vi "Process.vi"(11 "Actor":refnum<class "Status Window.lvclass">) -> ()   [LabVIEW 2015, in "Status Window.lvclass"]
uses:
  Status Window.lvclass
  Re-use Libraries/Minimal Actor Framework/Actors/Base Actor/Actor/Front Panel State.ctl
  Re-use Libraries/Minimal Actor Framework/Actors/Base Actor/Actor/Actor.lvclass
  Re-use Libraries/Minimal Actor Framework/Messaging/Message/Message.lvclass
  Actors/Alarm Handler/API/Alarm Handler Actor API.lvclass
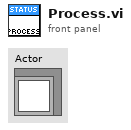
[diagram p1: front panel]
types:
  T1 = typedef "Actor.lvclass/Front Panel State.ctl" = enum32{"Invalid", "Standard", "Closed", "Hidden", "Minimized", "Maximized"}
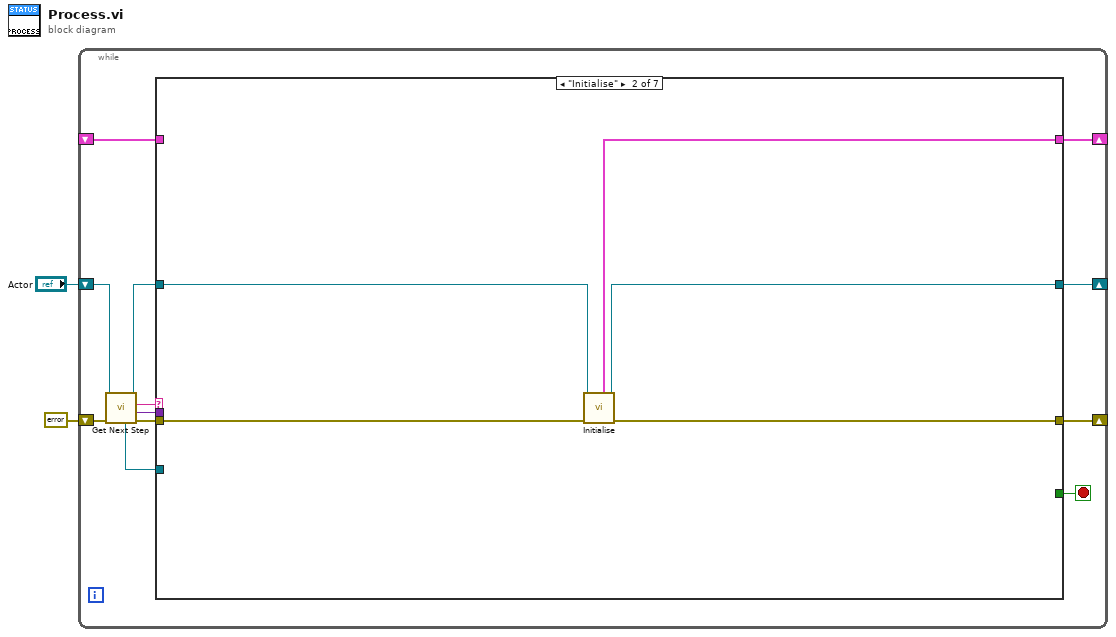
[diagram p0: block diagram]
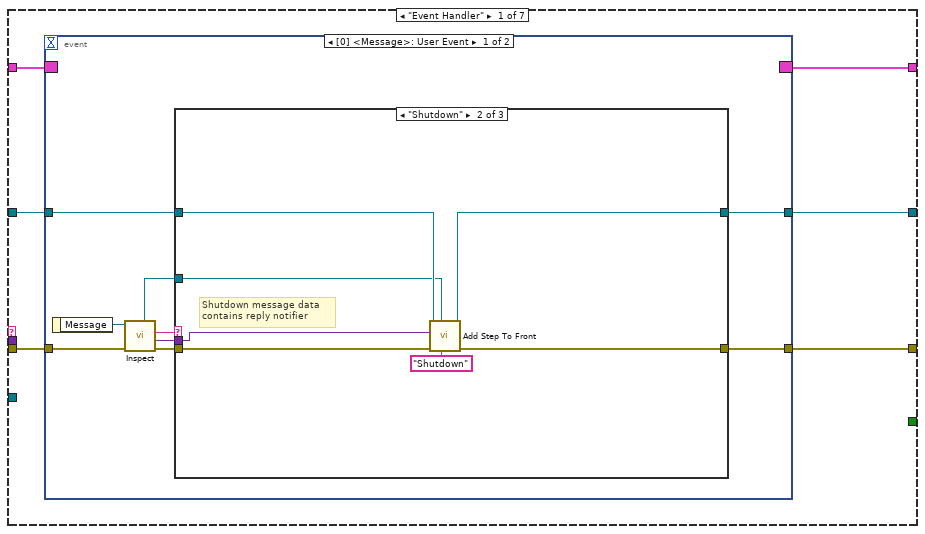
[diagram p2: hidden frame]
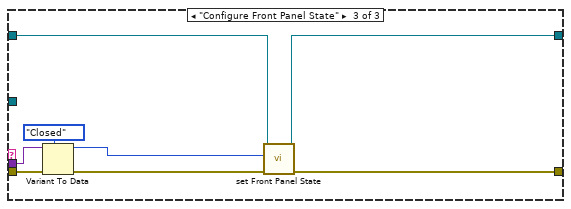
[diagram p4: hidden frame]
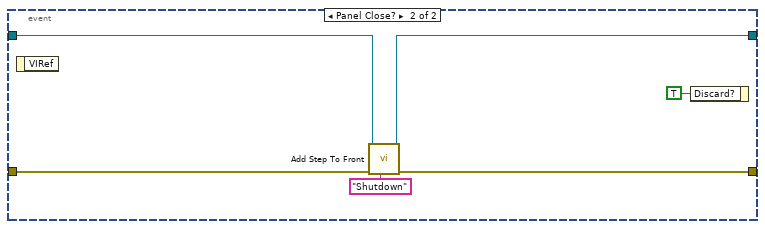
[diagram p5: hidden frame]
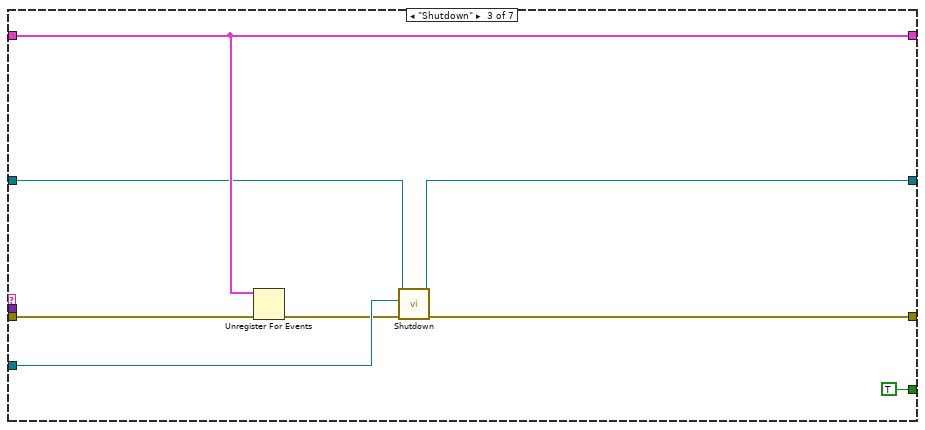
[diagram p6: hidden frame]
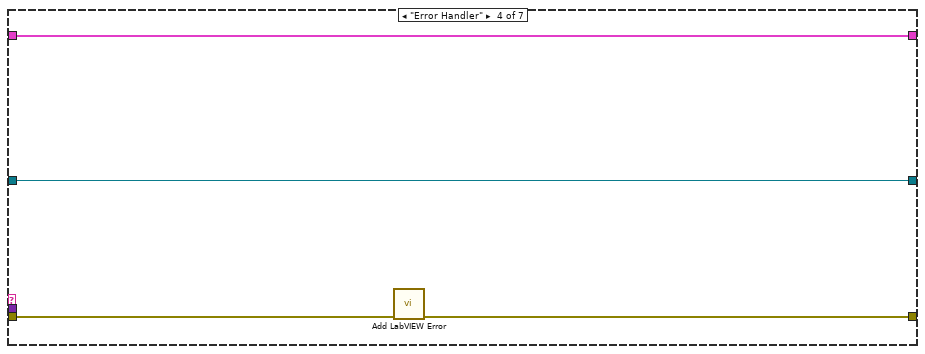
[diagram p7: hidden frame]
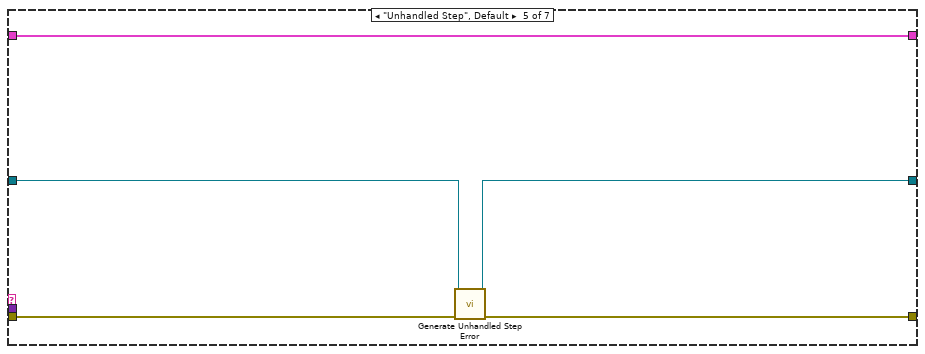
[diagram p8: hidden frame]
diagram:
  n1 = while {
    shift-right: [w5] -> _
    shift-left: "Actor" -> [w13]
    shift-right: [w10] -> _
    shift-left: _ -> [w9]
    shift-right: [w4] -> _
    shift-left: errorcluster {"status"=FALSE, "code"=0, "source"=""} ("error constant") -> [w7]
    stop <- w14 stop-if-true
    n2 = call-dynamic "Get Next Step.vi"("error in (no error)"=w7, "Actor in"=w13) -> ("error out"=w8:errorcluster, "Parameter"=w11:variant, "Step"=w6:string, "Actor out"=w12:refnum<class "Status Window.lvclass">, "Reply Channel"=w3:refnum<notifier>)  [unwired: 5 in]
    n3 = case shown="\"Initialise\"" w6 {
      tunnel: [_ _ TRUE _ _ _ _] -> w14
      tunnel: w12 -> [w20 w55 w63 w66 w73 w76 w78]
      tunnel: [w15 w53 w62 w66 w72 w76 w78] -> w5
      tunnel: w11 -> [_ _ _ _ _ _ _]
      tunnel: [w18 w57 w64 w69 w74 w77 w80] -> w10
      tunnel: w9 -> [w19 _ w64 w69 w74 w77 w80]
      tunnel: w8 -> [w17 w54 w60 w68 w71 w75 w79]
      tunnel: [w16 w56 w58 w67 w70 w75 w79] -> w4
      tunnel: w3 -> [_ _ w61 _ _ _ _]
      frame "Event Handler" {
        n4 = event shown="[0] <Message>: User Event" {
          selector: w19 -> [_ _]
          dyn-events: [_ _] -> w18
          timeout: _ -> [_ _]
          tunnel: w20 -> [w29 w48]
          tunnel: [w28 w47] -> w15
          tunnel: w17 -> [w26 w50]
          tunnel: [w27 w49] -> w16
          event User Event {
            n5 = event-data() -> ("Message"=w25:refnum<class "Message.lvclass">)  [unwired: 1 in]
            n6 = call "Inspect.vi"("error in (no error)"=w26, "Message in"=w25) -> ("error out"=w22:errorcluster, "Data"=w23:variant, "Name"=w24:string, "Reply Channel"=w21:refnum<notifier>)  [unwired: 5 in, 1 out]
            n7 = case shown="\"Shutdown\"" w24 {
              tunnel: w29 -> [w31 w38 w46]
              tunnel: [w31 w37 w45] -> w28
              tunnel: w22 -> [w30 w35 w42]
              tunnel: [w30 w34 w44] -> w27
              tunnel: w23 -> [_ w33 w43]
              tunnel: w21 -> [_ w32 _]
              frame Default {
              }
              frame "Shutdown" {
                # "Shutdown message data contains reply notifier"
                n8 = call-dynamic "Add Step To Front.vi"("Step Name"="Shutdown", "Reply Channel"=w32, "error in (no error)"=w35, "Parameter"=w33, "Actor in"=w38) -> ("error out"=w34:errorcluster, "Actor out"=w37:refnum<class "Status Window.lvclass">)  [unwired: 5 in]
              }
              frame "Configure Front Panel State" {
                n9 = Variant To Data(error in=w42, type=Front_Panel_State."Closed" ("Front Panel State"), Variant=w43) -> (data=w39:T1, error out=w41:errorcluster)
                n10 = call-dynamic "set Front Panel State.vi"("error in (no error)"=w41, "Front Panel State"=w39, "Actor in"=w46) -> ("error out"=w44:errorcluster, "Actor out"=w45:refnum<class "Status Window.lvclass">)  [unwired: 7 in]
              }
            }
          }
          event Panel Close? {
            n11 = event-data() -> ()  [unwired: 1 in, 1 out]
            n12 = call-dynamic "Add Step To Front.vi"("Step Name"="Shutdown", "error in (no error)"=w50, "Actor in"=w48) -> ("error out"=w49:errorcluster, "Actor out"=w47:refnum<class "Status Window.lvclass">)  [unwired: 7 in]
            n13 = event-data("Discard?"=TRUE) -> ()  [unwired: 1 in, 1 out]
          }
        }
      }
      frame "Initialise" {
        n14 = call "Initialise.vi"("error in (no error)"=w54, "Actor in"=w55) -> ("error out"=w56:errorcluster, "Actor out"=w53:refnum<class "Status Window.lvclass">, "Observers"=w57:cluster{"Actor":refnum<event-registration>})  [unwired: 7 in]
      }
      frame "Shutdown" {
        n15 = Unregister For Events(event registration refnum=w64, error in=w60) -> (error out=w59:errorcluster)
        n16 = call-dynamic "Shutdown.vi"("error in (no error)"=w59, "Reply Channel"=w61, "Actor in"=w63) -> ("error out"=w58:errorcluster, "Actor out"=w62:refnum<class "Status Window.lvclass">)  [unwired: 7 in]
      }
      frame "Error Handler" {
        n17 = call "Add LabVIEW Error.vi"("error in (no error)"=w68) -> ("error out"=w67:errorcluster)  [unwired: 10 in]
      }
      frame "Unhandled Step", Default {
        n18 = call-dynamic "Generate Unhandled Step Error.vi"("error in (no error)"=w71, "Actor in"=w73) -> ("error out"=w70:errorcluster, "Actor out"=w72:refnum<class "Status Window.lvclass">)  [unwired: 8 in]
      }
      frame "-----------------------" {
        # "Separator"
      }
      frame "Update State" {
        # "Not used"
      }
    }
  }
